vi "Dialog Box.vi"(8 "error in":errorcluster) -> (0 "error out":errorcluster, 1 "VISA Config Out":T1={"VISA Resource Name"="", "baud rate"=2400, "data bits"=7, "parity"=2, "stop bits"=10, "flow control"=0, "delay before read (ms) 2"=500, "Write Buffer"="Q\r\n"} {"flow control" items=["None"=0, "XON/XOFF"=1, "RTS/CTS"=2, "DTR/DSR"=4]; "stop bits" items=["1.0"=10, "1.5"=15, "2.0"=20]; "parity" items=["None", "Odd", "Even", "Mark", "Space"]; "data bits" min=5 max=8 step=1}, 2 "NI DAQ Config Out":T2={"Physical Channels"="", "Number of Samples"=500, "Desired Sample Rate (Hz)"=5000.0, "Minimum Value"=0.0, "Maximum Value"=10.0, "Input Terminal Configuration"=10083, "Sample Mode"=10123, "DAQmx Task Name"=""} {"Sample Mode" items=["Finite Samples"=10178, "Continuous Samples"=10123, "Hardware Timed Single Point"=12522]; "Input Terminal Configuration" items=["Default"=-1, "RSE"=10083, "NRSE"=10078, "Differential"=10106, "Pseudodifferential"=12529]})   [LabVIEW 2021]
uses:
  ConfigNI.ctl
  ConfigVISA.ctl
panel:
  in  "Cancel":bool
  in  "Ok":bool
  in  "VISA Config":T1={"VISA Resource Name"="", "baud rate"=2400, "data bits"=7, "parity"=2, "stop bits"=10, "flow control"=0, "delay before read (ms) 2"=500, "Write Buffer"="Q\r\n"} {"flow control" items=["None"=0, "XON/XOFF"=1, "RTS/CTS"=2, "DTR/DSR"=4]; "stop bits" items=["1.0"=10, "1.5"=15, "2.0"=20]; "parity" items=["None", "Odd", "Even", "Mark", "Space"]; "data bits" min=5 max=8 step=1}
  in  "NI DAQ Config":T2={"Physical Channels"="", "Number of Samples"=500, "Desired Sample Rate (Hz)"=5000.0, "Minimum Value"=0.0, "Maximum Value"=10.0, "Input Terminal Configuration"=10083, "Sample Mode"=10123, "DAQmx Task Name"=""} {"Sample Mode" items=["Finite Samples"=10178, "Continuous Samples"=10123, "Hardware Timed Single Point"=12522]; "Input Terminal Configuration" items=["Default"=-1, "RSE"=10083, "NRSE"=10078, "Differential"=10106, "Pseudodifferential"=12529]}
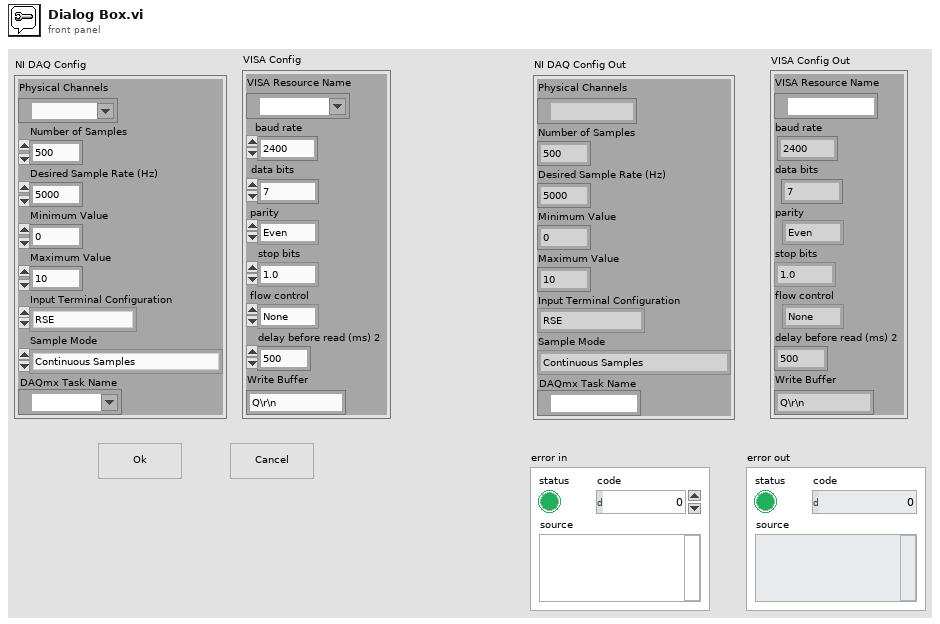
[diagram p1: front panel]
types:
  T1 = typedef "ConfigVISA.ctl" = cluster{"VISA Resource Name":refnum<visa-resource-name>, "baud rate":u32, "data bits":u16, "parity":u16, "stop bits":u16, "flow control":u16, "delay before read (ms) 2":u32, "Write Buffer":string}
  T2 = typedef "ConfigNI.ctl" = cluster{"Physical Channels":tag, "Number of Samples":i32, "Desired Sample Rate (Hz)":dbl, "Minimum Value":dbl, "Maximum Value":dbl, "Input Terminal Configuration":i32, "Sample Mode":i32, "DAQmx Task Name":refnum<k21>}
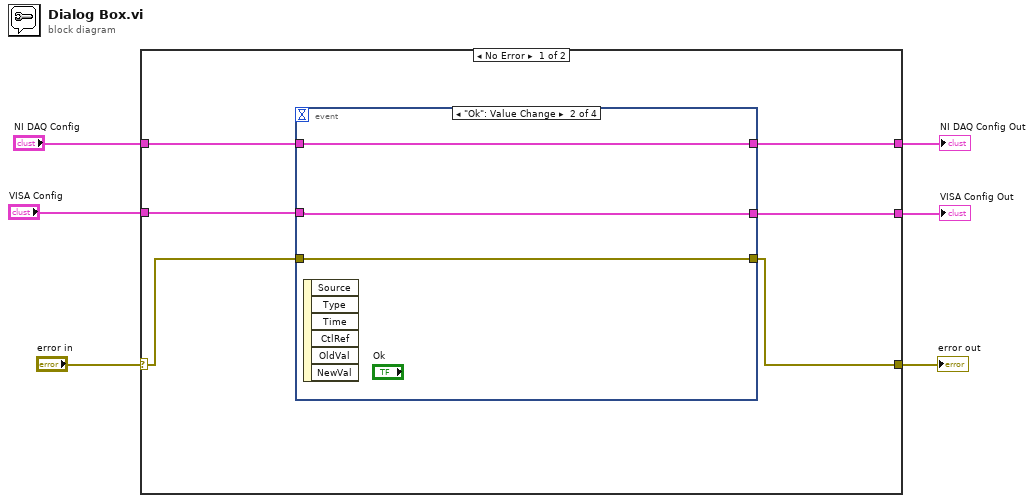
[diagram p0: block diagram]
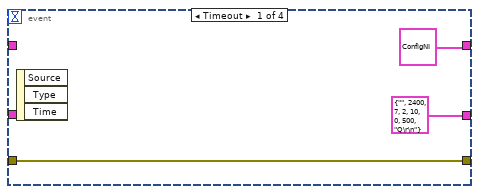
[diagram p2: hidden frame]
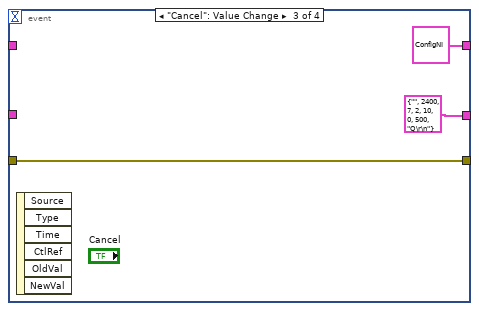
[diagram p3: hidden frame]
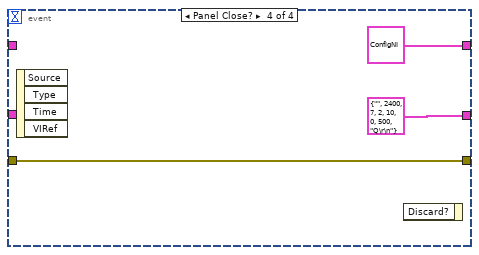
[diagram p4: hidden frame]
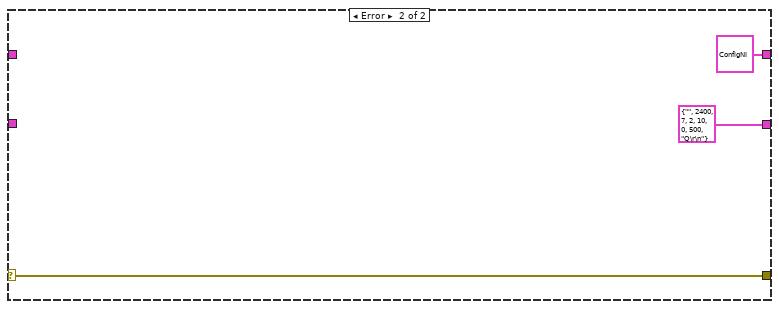
[diagram p5: hidden frame]
diagram:
  n1 = case shown="No Error" "error in" {
    selector: "error in" -> [w8 w27]
    tunnel: "NI DAQ Config" -> [w12 _]
    tunnel: "VISA Config" -> [w11 _]
    tunnel: [w7 w27] -> w3
    tunnel: [w10 T2 {"Physical Channels"="Dev6/ai0:1", "Number of Samples"=500, "Desired Sample Rate (Hz)"=5000.0, "Minimum Value"=0.0, "Maximum Value"=10.0, "Input Terminal Configuration"=10083, "Sample Mode"=10123, "DAQmx Task Name"=""} ("NI DAQ Config")] -> w2
    tunnel: [w9 T1 {"VISA Resource Name"="", "baud rate"=2400, "data bits"=7, "parity"=2, "stop bits"=10, "flow control"=0, "delay before read (ms) 2"=500, "Write Buffer"="Q\r\n"} ("VISA Config")] -> w1
    frame No Error {
      n2 = event shown="[1] \"Ok\": Value Change" {
        selector: _ -> [_ _ _ _]
        dyn-events: _ -> [_ _ _ _]
        timeout: _ -> [_ _ _ _]
        tunnel: w12 -> [_ w18 _ _]
        tunnel: w11 -> [_ w17 _ _]
        tunnel: [T2 {"Physical Channels"="Dev6/ai0:1", "Number of Samples"=500, "Desired Sample Rate (Hz)"=5000.0, "Minimum Value"=0.0, "Maximum Value"=10.0, "Input Terminal Configuration"=10083, "Sample Mode"=10123, "DAQmx Task Name"=""} ("NI DAQ Config") w18 T2 {"Physical Channels"="Dev6/ai0:1", "Number of Samples"=500, "Desired Sample Rate (Hz)"=5000.0, "Minimum Value"=0.0, "Maximum Value"=10.0, "Input Terminal Configuration"=10083, "Sample Mode"=10123, "DAQmx Task Name"=""} ("NI DAQ Config") T2 {"Physical Channels"="Dev6/ai0:1", "Number of Samples"=500, "Desired Sample Rate (Hz)"=5000.0, "Minimum Value"=0.0, "Maximum Value"=10.0, "Input Terminal Configuration"=10083, "Sample Mode"=10123, "DAQmx Task Name"=""} ("NI DAQ Config")] -> w10
        tunnel: [T1 {"VISA Resource Name"="", "baud rate"=2400, "data bits"=7, "parity"=2, "stop bits"=10, "flow control"=0, "delay before read (ms) 2"=500, "Write Buffer"="Q\r\n"} ("VISA Config") w17 T1 {"VISA Resource Name"="", "baud rate"=2400, "data bits"=7, "parity"=2, "stop bits"=10, "flow control"=0, "delay before read (ms) 2"=500, "Write Buffer"="Q\r\n"} ("VISA Config") T1 {"VISA Resource Name"="", "baud rate"=2400, "data bits"=7, "parity"=2, "stop bits"=10, "flow control"=0, "delay before read (ms) 2"=500, "Write Buffer"="Q\r\n"} ("VISA Config")] -> w9
        tunnel: [w13 w16 w19 w22] -> w7
        tunnel: w8 -> [w13 w16 w19 w22]
        event Timeout {
          n3 = event-data() -> ()  [unwired: 1 in, 3 out]
        }
        event "Ok": Value Change {
          n4 = event-data() -> ()  [unwired: 1 in, 6 out]
        }
        event "Cancel": Value Change {
          n5 = event-data() -> ()  [unwired: 1 in, 6 out]
        }
        event Panel Close? {
          n6 = event-data() -> ()  [unwired: 1 in, 4 out]
          n7 = event-data() -> ()  [unwired: 2 in, 1 out]
        }
      }
    }
    frame Error {
    }
  }
  "VISA Config Out" <- w1
  "NI DAQ Config Out" <- w2
  "error out" <- w3
